vi "stop.vi"(8 "error in (no error)":errorcluster, 9 "CameraSettings":refnum<class "CamaraSettings.lvclass">, 10 "stop":bool, 11 "Camera in":refnum<class "Camera.lvclass">) -> (0 "error out":errorcluster, 1 "imageSaved":bool, 2 "stopped?":bool, 3 "Camera out":refnum<class "Camera.lvclass">)   [LabVIEW 2009, in "Hardware.lvlib" / "Channels.lvlib" / "Camera.lvclass"]
uses:
  Camera.lvclass
  Tools/CameraSettings/CamaraSettings.lvclass
  Camera.lvclass/Camera.ctl
  Tools/Filing/FileSystem/FileSystem.lvclass
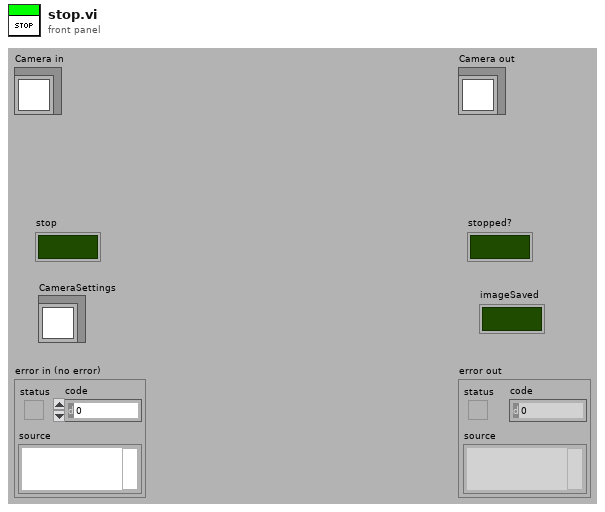
[diagram p1: front panel]
types:
  T1 = cluster{"cameraType":string, "imageName":string, "saved":string, "analysisType":string, "I16bit image data":i16[][], "path":path}
  T2 = typedef "Image Type" = u32
  T3 = typedef "IMAQ Image.ctl" = refnum<image>
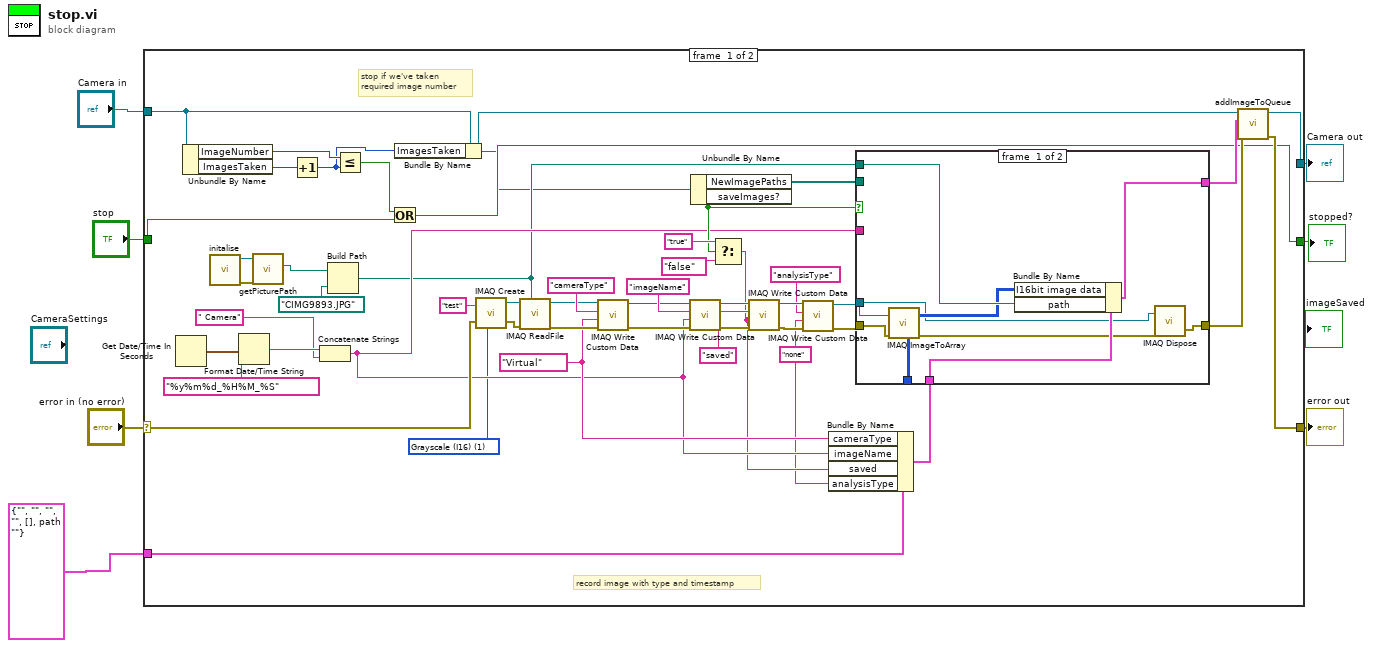
[diagram p0: block diagram]
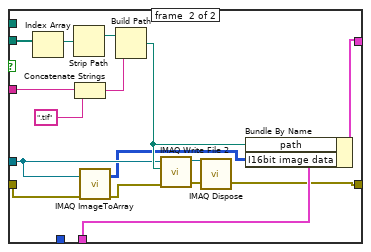
[diagram p2: hidden frame]
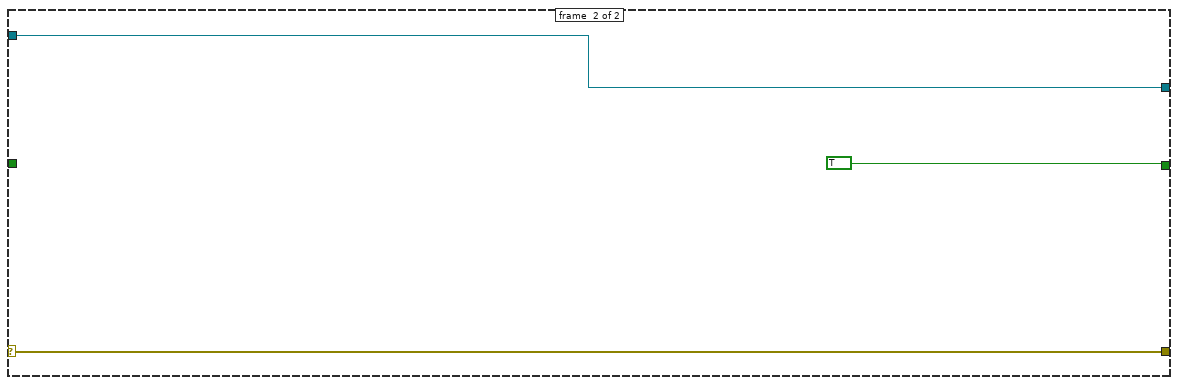
[diagram p3: hidden frame]
diagram:
  n1 = case shown="No Error" "error in (no error)" {
    selector: "error in (no error)" -> [w55 w85]
    tunnel: [w53 w85] -> w6
    tunnel: [w54 w84] -> w4
    tunnel: "Camera in" -> [w11 w84]
    tunnel: [w12 TRUE] -> w3
    tunnel: "stop" -> [w13 _]
    tunnel: T1 {"cameraType"="", "imageName"="", "saved"="", "analysisType"="", "I16bit image data"=[], "path"=path ""} ("ImageData") -> [w24 _]
    frame #0 {
      w8 = T2 1 items=["Grayscale (U8)", "Grayscale (I16)", "Grayscale (SGL)", "Complex (CSG)", "RGB (U32)", "HSL (U32)", "RGB (U64)", "Grayscale (U16)"] ("Image Type")
      w20 = "none"
      w23 = "Virtual"
      # "stop if we've taken \nrequired image number"
      # "record image with type and timestamp"
      n2 = Get Date/Time In Seconds() -> (seconds since 1Jan1904=w47:timestamp)
      n3 = Unbundle By Name(w11) -> ("ImageNumber"=w15:i32, "ImagesTaken"=w16:i32)
      n4 = call "initalise.vi"() -> ("error out"=w50:errorcluster, "FileSystem out"=w51:refnum<class "FileSystem.lvclass">)  [unwired: 10 in]
      n5 = Format Date/Time String(time format string (%c)="%y%m%d_%H%M_%S", seconds (now)=w47) -> (date/time string=w45:string)  [unwired: 1 in]
      n6 = call "getPicturePath.vi"("error in (no error)"=w50, "FileSystem in"=w51) -> ("PicturePath"=w49:path)  [unwired: 7 in, 2 out]
      n7 = Increment(x=w16) -> (x+1=w9:i32)
      n8 = Concatenate Strings(w45, " Camera") -> (w22:string)
      n9 = Build Path(base path=w49, name or relative path=path "CIMG9893.JPG" ("File Path")) -> (appended path=w17:path)
      n10 = Less Or Equal?(x=w15, y=w9) -> (x <= y?=w14:bool)
      n11 = Or(x=w14, y=w13) -> (x .or. y?=w12:bool)
      n12 = Bundle By Name(cluster=w11, "ImagesTaken"=w9) -> (w10:refnum<class "Camera.lvclass">)
      n13 = call "IMAQ Create"("Image Name"="test", "Image Type"=w8, "error in (no error)"=w55) -> ("New Image"=w57:T3, "error out"=w56:errorcluster)  [unwired: 2 in]
      n14 = call "IMAQ ReadFile"("File Path"=w17, "error in (no error)"=w56, "Image"=w57) -> ("error out"=w40:errorcluster, "Image Out"=w41:T3)  [unwired: 4 in, 3 out]
      n15 = call "IMAQ Write Custom Data"("error in (no error)"=w40, "Custom Data In"=w23, "Key"="cameraType", "Image"=w41) -> ("error out"=w38:errorcluster, "Image Out"=w39:T3)  [unwired: 6 in]
      n16 = call "IMAQ Write Custom Data"("error in (no error)"=w38, "Custom Data In"=w22, "Key"="imageName", "Image"=w39) -> ("error out"=w36:errorcluster, "Image Out"=w37:T3)  [unwired: 6 in]
      n17 = Unbundle By Name(w10) -> ("NewImagePaths"=w33:path[], "saveImages?"=w30:bool)
      n18 = Select(t="true", s=w30, f="false") -> (s? t:f=w21:string)
      n19 = call "IMAQ Write Custom Data"("error in (no error)"=w36, "Custom Data In"=w21, "Key"="saved", "Image"=w37) -> ("error out"=w28:errorcluster, "Image Out"=w29:T3)  [unwired: 6 in]
      n20 = call "IMAQ Write Custom Data"("error in (no error)"=w28, "Custom Data In"=w20, "Key"="analysisType", "Image"=w29) -> ("error out"=w27:errorcluster, "Image Out"=w26:T3)  [unwired: 6 in]
      n21 = Bundle By Name(cluster=w24, "cameraType"=w23, "imageName"=w22, "saved"=w21, "analysisType"=w20) -> (w19:T1)
      n22 = case shown="False" w30 {
        tunnel: w27 -> [w63 w72]
        tunnel: [w61 w67] -> w34
        tunnel: w26 -> [w60 w71]
        tunnel: [w65 w75] -> w18
        tunnel: w33 -> [_ w82]
        tunnel: w22 -> [_ w79]
        tunnel: w19 -> [w66 w76]
        tunnel: w17 -> [w64 _]
        tunnel: [w58 _] -> _
        frame #0 {
          n23 = call "IMAQ ImageToArray"("error in (no error)"=w63, "Image"=w60) -> ("Image Pixels (U16)"=w58:u16[][], "error out"=w59:errorcluster, "Image Pixels (I16)"=w62:i16[][])  [unwired: 2 in, 2 out]
          n24 = Bundle By Name(cluster=w66, "I16bit image data"=w62, "path"=w64) -> (w65:T1)
          n25 = call "IMAQ Dispose"("Image"=w60, "error in (no error)"=w59) -> ("error out"=w61:errorcluster)  [unwired: 4 in]
        }
        frame #1 {
          n26 = Index Array(array=w82) -> (element=w81:path)  [unwired: 1 in]
          n27 = Strip Path(path=w81) -> (stripped path=w80:path)  [unwired: 1 out]
          n28 = Concatenate Strings(w79, ".tif") -> (w77:string)
          n29 = call "IMAQ ImageToArray"("error in (no error)"=w72, "Image"=w71) -> ("error out"=w73:errorcluster, "Image Pixels (I16)"=w70:i16[][])  [unwired: 2 in, 3 out]
          n30 = Build Path(base path=w80, name or relative path=w77) -> (appended path=w74:path)
          n31 = call-poly "IMAQ Write File 2"("error in (no error)"=w73, "File Path"=w74, "Image"=w71) -> ("error out"=w68:errorcluster, "Image Out (duplicate)"=w69:T3)  [unwired: 7 in]
          n32 = call "IMAQ Dispose"("Image"=w69, "error in (no error)"=w68) -> ("error out"=w67:errorcluster)  [unwired: 4 in]
          n33 = Bundle By Name(cluster=w76, "path"=w74, "I16bit image data"=w70) -> (w75:T1)
        }
      }
      n34 = call "addImageToQueue.vi"("error in (no error)"=w34, "ImageData"=w18, "Camera in"=w10) -> ("error out"=w53:errorcluster, "Camera out"=w54:refnum<class "Camera.lvclass">)  [unwired: 7 in]
    }
    frame #1 {
    }
  }
  "error out" <- w6
  "Camera out" <- w4
  "stopped?" <- w3
